vi "PAS_set_DAC.vi"(8 "error in (no error)":errorcluster, 9 "Voltage":dbl, 10 "Channel":u16(ring) items=["CH 1"=1, "CH 2"=2, "BOTH"=3], 11 "VISA Refnum in":refnum<visa-resource-name>) -> (0 "error out":errorcluster, 1 "Success?":bool, 3 "VISA Refnum out":refnum<visa-resource-name>)   [LabVIEW 2020]
panel:
  out "decimal integer string":string
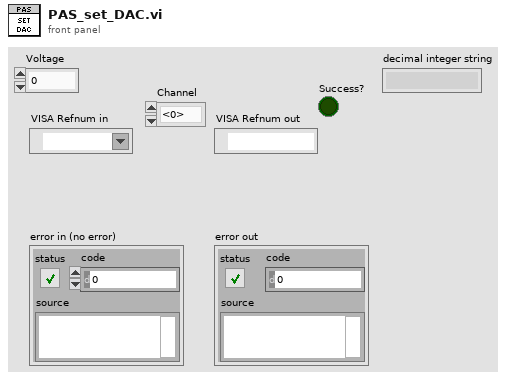
[diagram p1: front panel]
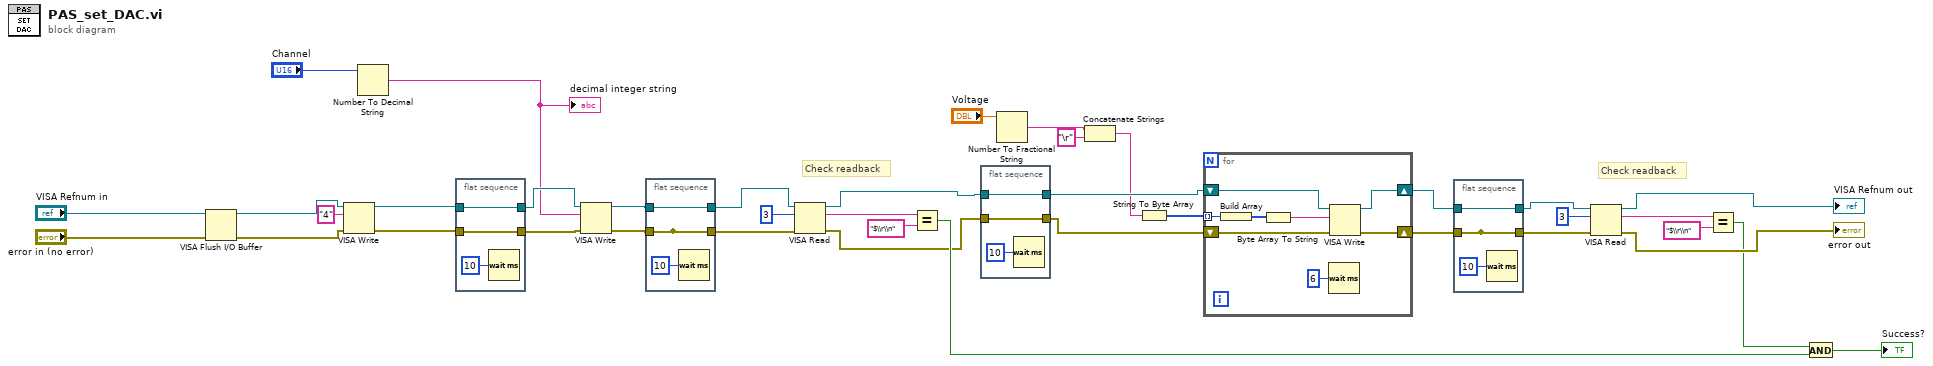
[diagram p0: block diagram]
diagram:
  # "Check readback"
  # "Check readback"
  n1 = VISA Flush I/O Buffer(VISA resource name="VISA Refnum in", error in (no error)="error in (no error)") -> (VISA resource name out=w18:refnum<visa-resource-name>, error out=w16:errorcluster)  [unwired: 1 in]
  n2 = VISA Write(VISA resource name=w18, write buffer="4", error in (no error)=w16) -> (VISA resource name out=w36:refnum<visa-resource-name>, error out=w37:errorcluster)  [unwired: 1 out]
  n3 = Number To Decimal String(number="Channel") -> (decimal integer string=w33:string)  [unwired: 1 in]
  "decimal integer string" <- w33
  n4 = flat-sequence {
    tunnel: w36 -> [w41]
    tunnel: [w41] -> w38
    tunnel: w37 -> [w40]
    tunnel: [w40] -> w39
    frame #0 {
      n5 = Wait (ms)(milliseconds to wait=u32 10) -> ()  [unwired: 1 out]
    }
  }
  n6 = VISA Write(VISA resource name=w38, write buffer=w33, error in (no error)=w39) -> (VISA resource name out=w6:refnum<visa-resource-name>, error out=w8:errorcluster)  [unwired: 1 out]
  n7 = flat-sequence {
    tunnel: w6 -> [w44]
    tunnel: [w44] -> w5
    tunnel: [w43] -> _
    tunnel: [w43] -> w7
    tunnel: w8 -> [w43]
    frame #0 {
      n8 = Wait (ms)(milliseconds to wait=u32 10) -> ()  [unwired: 1 out]
    }
  }
  n9 = VISA Read(VISA resource name=w5, byte count=u32 3, error in (no error)=w7) -> (VISA resource name out=w15:refnum<visa-resource-name>, read buffer=w31:string, error out=w13:errorcluster)  [unwired: 1 out]
  n10 = Equal?(x=w31, y="$\\r\\n") -> (x = y?=w29:bool)
  n11 = flat-sequence {
    tunnel: w15 -> [w47]
    tunnel: [w47] -> w14
    tunnel: w13 -> [w46]
    tunnel: [w46] -> w12
    frame #0 {
      n12 = Wait (ms)(milliseconds to wait=u32 10) -> ()  [unwired: 1 out]
    }
  }
  n13 = Number To Fractional String(number="Voltage") -> (F-format string=w11:string)  [unwired: 3 in]
  n14 = Concatenate Strings(w11, "\r" ("string")) -> (w10:string)
  n15 = String To Byte Array(string=w10) -> (unsigned byte array=w20:u8[])
  n16 = for {
    tunnel: w20 -> [w52] mode=indexing
    shift-right: [w55] -> w2
    shift-left: w14 -> [w54]
    shift-right: [w56] -> w4
    shift-left: w12 -> [w53]
    n17 = Build Array(w52) -> (w51:u8[])
    n18 = Byte Array To String(unsigned byte array=w51) -> (string=w50:string)
    n19 = Wait (ms)(milliseconds to wait=u32 6) -> ()  [unwired: 1 out]
    n20 = VISA Write(VISA resource name=w54, write buffer=w50, error in (no error)=w53) -> (VISA resource name out=w55:refnum<visa-resource-name>, error out=w56:errorcluster)  [unwired: 1 out]
  }
  n21 = flat-sequence {
    tunnel: w2 -> [w57]
    tunnel: [w57] -> w1
    tunnel: [w58] -> _
    tunnel: [w58] -> w3
    tunnel: w4 -> [w58]
    frame #0 {
      n22 = Wait (ms)(milliseconds to wait=u32 10) -> ()  [unwired: 1 out]
    }
  }
  n23 = VISA Read(VISA resource name=w1, byte count=u32 3, error in (no error)=w3) -> (VISA resource name out=→"VISA Refnum out":refnum<visa-resource-name>, read buffer=w27:string, error out=→"error out":errorcluster)  [unwired: 1 out]
  n24 = Equal?(x=w27, y="$\\r\\n") -> (x = y?=w21:bool)
  n25 = And(x=w21, y=w29) -> (x .and. y?=→"Success?":bool)
